vi "IQ_to_RF.vi"(7 "Header In":T1={"header info"={"Header"="", "Head length"=0}, "A/D info"={"# rf points per line"=0, "# lines per scan"=0, "sample rate MHz"=0, "# A/D bits"=0, "# bytes per A/D"=0, "TGC Flag"=0, "A/D Type"=""}, "Tranducer Info"={"bandwidth"=0.0, "center freq"=0.0, "start freq"=0.0, "ID"=0}, "Scan Info"={"delay"=0.0, "pivot distance"=0.0, "sector scan angle"=0.0, "operator"="", "Scan Mode"="", "location"=""}, "Time/Date Info"={"date"="", "time"=""}, "RF Info"={"RF file name"="", "RF file att"="", "RF cal file name"="", "RF cal file att"=""}, "Patient Info"={"ID"="", "extended ID"="", "age"=0, "sex"="", "previously\nscanned"="", "PSA"=0.0, "LOS"=1, "Ethnicty 2"=3, "Race"=3}, "Tissue Type"={"organ"=0, "disease type"=0, "disease location"=0, "IQ_pts"=0, "RcvBuffer"=0, "RcvFrame"=0, "IQBuff"=0, "IQFrame"=0, "IQPage"=0}, "Votage scaling"={"Digitizer (dB)"=0.0, "Gain (dB)"=0.0, "Atten (dB)"=0.0}, "Comment"="", "Misc Info"={"avg num"=0, "c speed"=0, "Div By or SF zones"=0, "XMIT CHS"=0, "RCV CHS"=0, "Xmit angle"=0.0}, "Therapy Parameters"={"Theraputic Freq (MHz)"=0.1, "Time on (s)"=1.0, "Therapy amplitude (mV)"=50.0, "Lines Before"=20, "Lines After"=80}, "Scan Settings"={"Energy (uJ or V)"=0, "Damp (Ohm) or Fc"=0, "HP Filt (KHz)"=0, "LP Filt (MHz)"=0, "Gain (db)"=0, "prf (kHz)"=0.0, "Distance between\nscan lines (um)"=0, "Distance between\nscan planes (um)"=0, "Scan line gap (um)"=0.0, "Scan plane gap (um)"=0.0}, "Compression Parameters"={"F1 (MHz)"=0.0, "F2 (MHz)"=0.0, "% taper"=0.0, "duration"=0.0}, "Patient Info Xtra"={"First Name"="", "Last Name"="", "Notes"=""}, "ROI Box"=[]} {"Compression Parameters"."% taper" min=50 max=1000 format="%.2f"; "Compression Parameters"."F2 (MHz)" format="%.3f"; "Compression Parameters"."F1 (MHz)" format="%.3f"; "Scan Settings"."prf (kHz)" format="%.2f"; "Therapy Parameters"."Therapy amplitude (mV)" min=50 max=1000 format="%.2f"; "Therapy Parameters"."Time on (s)" format="%.3f"; "Therapy Parameters"."Theraputic Freq (MHz)" format="%.3f"; "Patient Info"."Race" items=["Am Ind or Alaska", "Asian", "Hawaiian, Pac Isl", "Black or Afr Amer", "White", "more than one race", "unknown"]; "Patient Info"."Ethnicty 2" items=["Hispanic", "Non-Hispanic", "unknown"]; "Patient Info"."LOS" items=["1", "2", "3", "4", "5"]; "Patient Info"."PSA" format="%.1f"; "Scan Info"."delay" format="%.2f"; "Scan Info"."pivot distance" format="%.2f"; "Scan Info"."sector scan angle" format="%.2f"; "Tranducer Info"."bandwidth" format="%.2f"; "Tranducer Info"."center freq" format="%.2f"; "Tranducer Info"."start freq" format="%.2f"}, 9 "IQ Array In":i32[](array[numeric]), 11 "IQ Array":csg[][](array[numeric])) -> (0 "Z Out":csg[][](array[numeric]), 3 "RF Array":sgl[][](array[numeric]))   [LabVIEW 2022 SP3]
uses:
  Header.ctl
  <vilib>/Analysis/2dsp.llb/Rational Resample (single channel, DBL).vi
  <vilib>/Analysis/NI_AALPro.lvlib
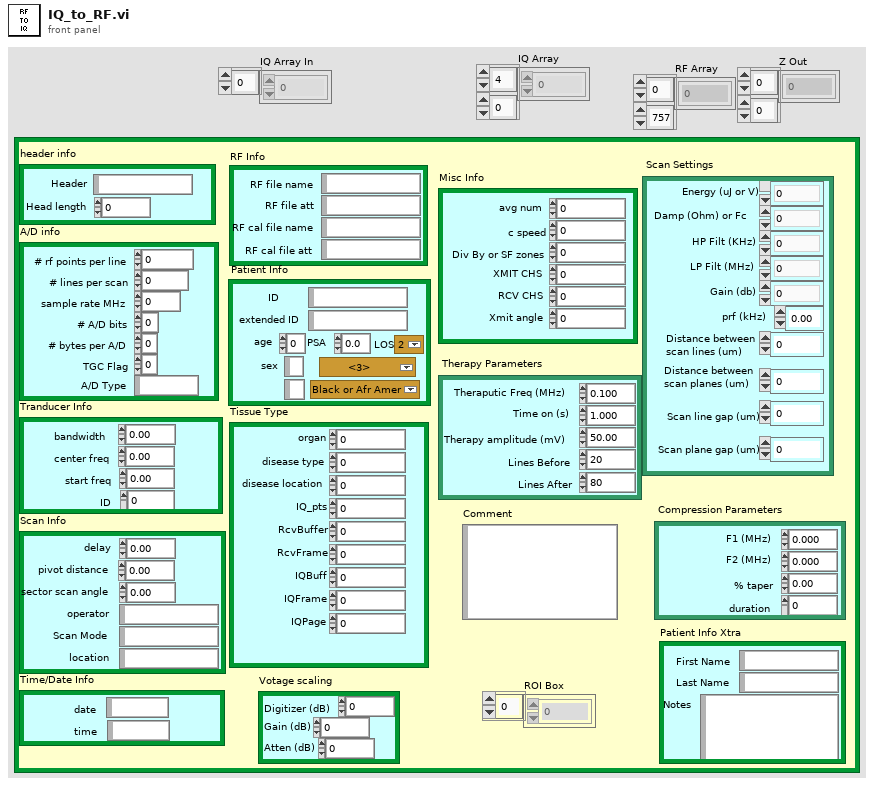
[diagram p1: front panel]
types:
  T1 = typedef "Header.ctl" = cluster{"header info":cluster{"Header":string, "Head length":i16}, "A/D info":cluster{"# rf points per line":u16, "# lines per scan":u16, "sample rate MHz":u16, "# A/D bits":i16, "# bytes per A/D":u16, "TGC Flag":u16, "A/D Type":string}, "Tranducer Info":cluster{"bandwidth":sgl, "center freq":sgl, "start freq":sgl, "ID":i32}, "Scan Info":cluster{"delay":sgl, "pivot distance":sgl, "sector scan angle":sgl, "operator":string, "Scan Mode":string, "location":string}, "Time/Date Info":cluster{"date":string, "time":string}, "RF Info":cluster{"RF file name":string, "RF file att":string, "RF cal file name":string, "RF cal file att":string}, "Patient Info":cluster{"ID":string, "extended ID":string, "age":u16, "sex":string, "previously\nscanned":string, "PSA":sgl, "LOS":u8, "Ethnicty 2":u8, "Race":u8}, "Tissue Type":cluster{"organ":i16, "disease type":i16, "disease location":i16, "IQ_pts":u16, "RcvBuffer":u8, "RcvFrame":u16, "IQBuff":u8, "IQFrame":u16, "IQPage":u8}, "Votage scaling":cluster{"Digitizer (dB)":sgl, "Gain (dB)":sgl, "Atten (dB)":sgl}, "Comment":string, "Misc Info":cluster{"avg num":u16, "c speed":i16, "Div By or SF zones":i16, "XMIT CHS":u8, "RCV CHS":u8, "Xmit angle":sgl}, "Therapy Parameters":cluster{"Theraputic Freq (MHz)":sgl, "Time on (s)":sgl, "Therapy amplitude (mV)":sgl, "Lines Before":u16, "Lines After":u16}, "Scan Settings":cluster{"Energy (uJ or V)":u8, "Damp (Ohm) or Fc":u8, "HP Filt (KHz)":u8, "LP Filt (MHz)":u8, "Gain (db)":u8, "prf (kHz)":sgl, "Distance between\nscan lines (um)":u16, "Distance between\nscan planes (um)":u16, "Scan line gap (um)":sgl, "Scan plane gap (um)":sgl}, "Compression Parameters":cluster{"F1 (MHz)":sgl, "F2 (MHz)":sgl, "% taper":sgl, "duration":sgl}, "Patient Info Xtra":cluster{"First Name":string, "Last Name":string, "Notes":string}, "ROI Box":u16[]}
  T2 = cluster{"alias rejection (dB)":dbl, "normalized bandwidth":dbl}
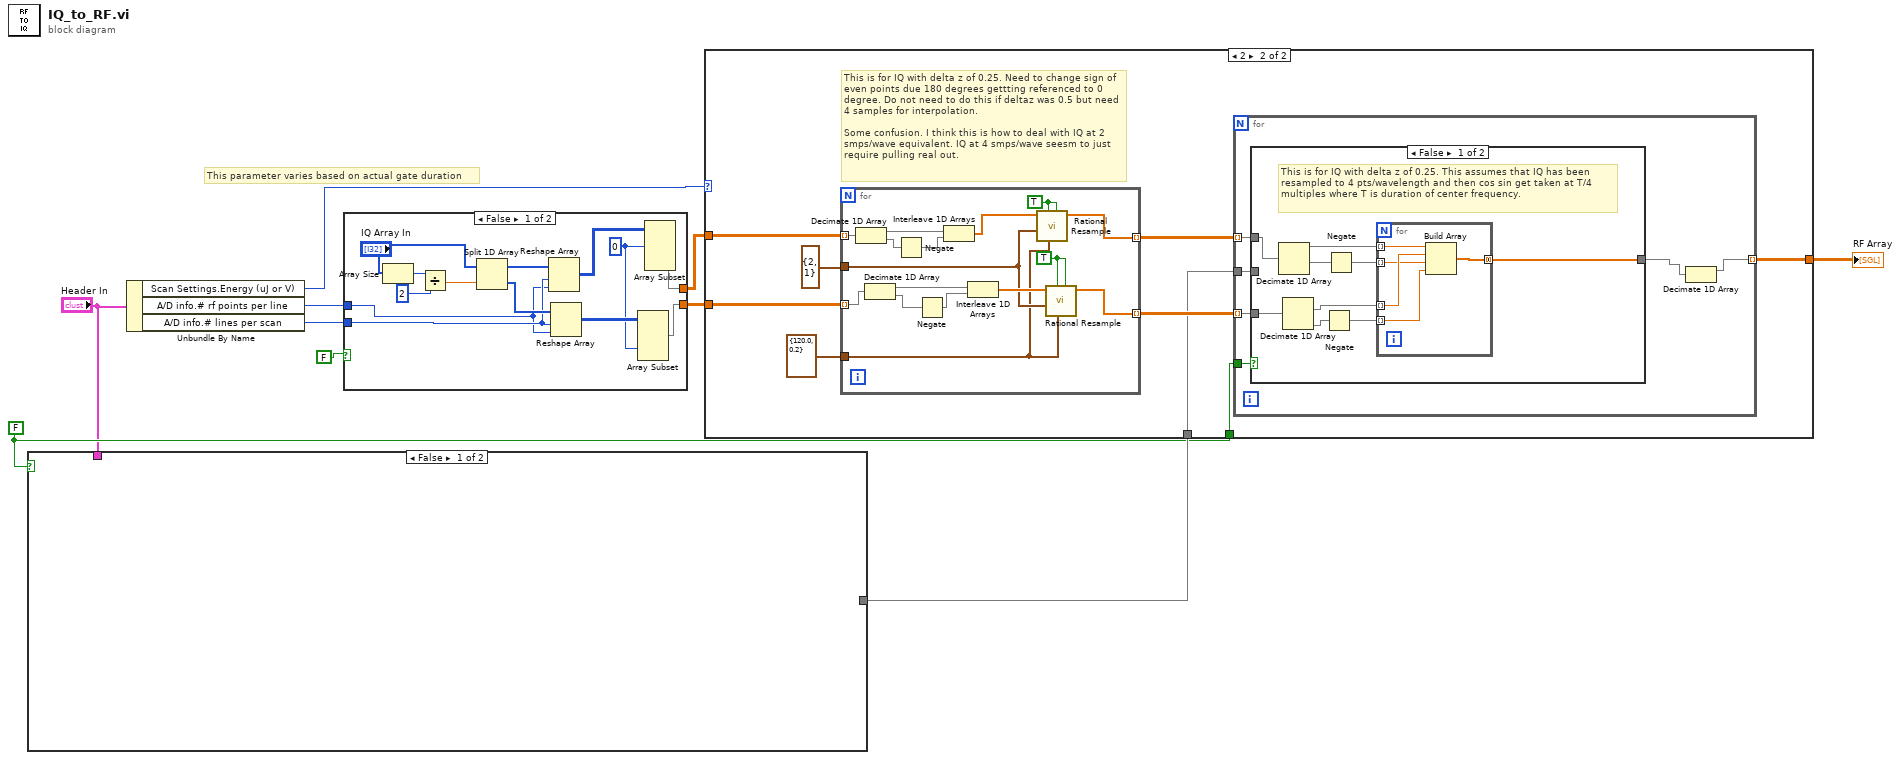
[diagram p0: block diagram]
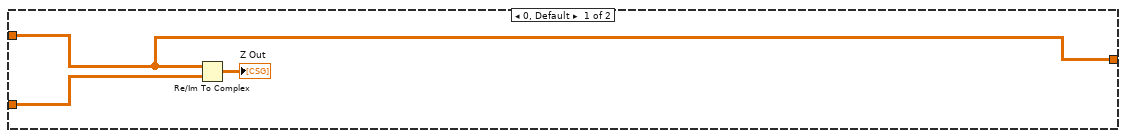
[diagram p2: hidden frame]
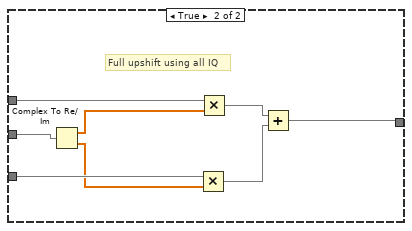
[diagram p3: hidden frame]
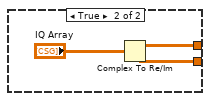
[diagram p4: hidden frame]
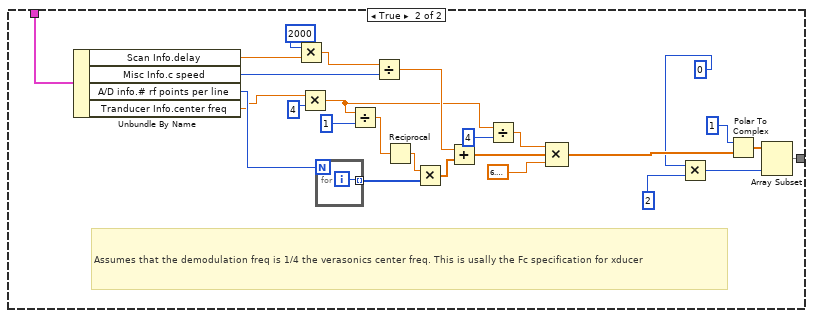
[diagram p5: hidden frame]
diagram:
  w9 = FALSE
  # "This parameter varies based on actual gate duration"
  n1 = case shown="False" w9 {
    tunnel: [_ w16] -> w10
    tunnel: "Header In" -> [_ w12]
    frame False {
    }
    frame True {
      # "Assumes that the demodulation freq is 1/4 the verasonics center freq. This is usally the Fc specification for xducer"
      n2 = Unbundle By Name(w12) -> ("Scan Info.delay"=w32:sgl, "Misc Info.c speed"=w29:i16, "A/D info.# rf points per line"=w33:u16, "Tranducer Info.center freq"=w15:sgl)
      n3 = Multiply(x=2000, y=w32) -> (x*y=w30:sgl)
      n4 = Multiply(x=w15, y=4) -> (x*y=w14:sgl)
      n5 = for {
        N: w33 -> [_]
        tunnel: [w37] -> w25 mode=indexing
        i -> [w37]
      }
      n6 = Divide(x=w14, y=1) -> (x/y=w24:sgl)
      n7 = Divide(x=w30, y=w29) -> (x/y=w28:sgl)
      n8 = Reciprocal(x=w24) -> (1/x=w23:sgl)
      n9 = Multiply(x=w23, y=w25) -> (x*y=w22:sgl[])
      n10 = Add(x=w28, y=w22) -> (x+y=w27:sgl[])
      n11 = Divide(x=w14, y=4) -> (x/y=w35:sgl)
      n12 = Compound Arithmetic op=MULTIPLY(w35, w27, 6.283185307179586) -> (w21:dbl[])
      n13 = Multiply(x=0 ("length"), y=2 ("upsampling factor")) -> (x*y=w17:i32)
      n14 = Polar To Complex(1:w21, 2:1 ("upsampling factor")) -> (0:w19:cdb[])
      n15 = Array Subset(array=w19, length=w17) -> (w16:cdb[])  [unwired: 1 in]
    }
  }
  n16 = Unbundle By Name("Header In") -> ("Scan Settings.Energy (uJ or V)"=w2:u8, "A/D info.# rf points per line"=w6:u16, "A/D info.# lines per scan"=w3:u16)
  n17 = case shown="False" FALSE {
    tunnel: w6 -> [w42 _]
    tunnel: [w46 w52] -> w5
    tunnel: [w44 w51] -> w4
    tunnel: w3 -> [w48 _]
    frame False {
      w43 = 0 ("index")
      n18 = Array Size(array="IQ Array In") -> (size(s)=w40:i32)
      n19 = Divide(x=w40, y=2) -> (x/y=w39:dbl)
      n20 = Split 1D Array(array="IQ Array In", index=w39) -> (first subarray=w50:i32[], second subarray=w49:i32[])
      n21 = Reshape Array(w50, w48, w42) -> (w47:i32[][])
      n22 = Reshape Array(w49, w48, w42) -> (w45:i32[][])
      n23 = Array Subset(array=w45, index (col)=w43) -> (w44:i32[][])  [unwired: 3 in]
      n24 = Array Subset(array=w47, index (col)=w43) -> (w46:i32[][])  [unwired: 3 in]
    }
    frame True {
      n25 = Complex To Re/Im(x + iy="IQ Array") -> (x=w52:sgl[][], y=w51:sgl[][])
    }
  }
  n26 = case shown="2" w2 {
    tunnel: w10 -> [_ w63]
    tunnel: w9 -> [_ w62]
    tunnel: w5 -> [w54 w61]
    tunnel: w4 -> [w56 w60]
    tunnel: [w54 w59] -> w1
    frame 0, Default {
      n27 = Re/Im To Complex(1:w56, 2:w54) -> (0:→"Z Out":csg[][])
    }
    frame 2 {
      # "This is for IQ with delta z of 0.25. Need to change sign of even points due 180 degrees gettting referenced to 0 degree. Do not need to do this if deltaz was 0.5 but need 4 samples for interpolation.\n\nSome confusion. I think this is how to deal with IQ at 2 smps/wave equivalent. IQ at 4 smps/wave seesm to just require pulling real out."
      n28 = for {
        tunnel: cluster{"interpolation":i32, "decimation":i32} {"interpolation"=2, "decimation"=1} ("resample factor") -> [w72]
        tunnel: w61 -> [w71] mode=indexing
        tunnel: w60 -> [w70] mode=indexing
        tunnel: T2 {"alias rejection (dB)"=120.0, "normalized bandwidth"=0.2} ("FIR filter specifications") -> [w69]
        tunnel: [w67] -> w65 mode=indexing
        tunnel: [w68] -> w64 mode=indexing
        w73 = TRUE ("anti-aliasing?")
        w78 = TRUE ("anti-aliasing?")
        n29 = Decimate 1D Array(w71) -> (w80:sgl[], w81:sgl[])
        n30 = Decimate 1D Array(w70) -> (w76:sgl[], w77:sgl[])
        n31 = Negate(x=w81) -> (-x=w79:sgl[])
        n32 = Negate(x=w77) -> (-x=w75:sgl[])
        n33 = Interleave 1D Arrays(w80, w79) -> (w66:sgl[])
        n34 = Interleave 1D Arrays(w76, w75) -> (w74:sgl[])
        n35 = call-poly <vilib>:"Rational Resample.vi"("anti-aliasing?"=w78, "FIR filter specifications"=w69, "reset"=w78, "resample factor"=w72, "X"=w66) -> ("Y"=w67:dbl[])  [unwired: 4 in, 2 out]
        n36 = call-poly <vilib>:"Rational Resample.vi"("anti-aliasing?"=w73, "FIR filter specifications"=w69, "reset"=w73, "resample factor"=w72, "X"=w74) -> ("Y"=w68:dbl[])  [unwired: 4 in, 2 out]
      }
      n37 = for {
        tunnel: [w82] -> w59 mode=indexing
        tunnel: w65 -> [w87] mode=indexing
        tunnel: w64 -> [w86] mode=indexing
        tunnel: w62 -> [w85]
        tunnel: w63 -> [w84]
        n38 = case shown="False" w85 {
          tunnel: [w93 w105] -> w83
          tunnel: w87 -> [w89 w109]
          tunnel: w86 -> [w88 w108]
          tunnel: w84 -> [_ w104]
          frame False {
            # "This is for IQ with delta z of 0.25. This assumes that IQ has been resampled to 4 pts/wavelength and then cos sin get taken at T/4 multiples where T is duration of center frequency."
            n39 = Decimate 1D Array(w89) -> (w96:dbl[], w92:dbl[])  [unwired: 2 out]
            n40 = Decimate 1D Array(w88) -> (w90:dbl[], w91:dbl[])  [unwired: 2 out]
            n41 = Negate(x=w91) -> (-x=w94:dbl[])
            n42 = Negate(x=w92) -> (-x=w95:dbl[])
            n43 = for {
              tunnel: w96 -> [w101] mode=indexing
              tunnel: w90 -> [w100] mode=indexing
              tunnel: w95 -> [w99] mode=indexing
              tunnel: w94 -> [w98] mode=indexing
              tunnel: [w97] -> w93 mode=concatenating
              n44 = Build Array(w101, w100, w99, w98) -> (w97:dbl[])
            }
          }
          frame True {
            # "Full upshift using all IQ"
            n45 = Complex To Re/Im(x + iy=w104) -> (x=w103:dbl[], y=w102:dbl[])
            n46 = Multiply(x=w108, y=w102) -> (x*y=w106:dbl[])
            n47 = Multiply(x=w109, y=w103) -> (x*y=w107:dbl[])
            n48 = Add(x=w107, y=w106) -> (x+y=w105:dbl[])
          }
        }
        n49 = Decimate 1D Array(w83) -> (w82:dbl[])  [unwired: 1 out]
      }
    }
  }
  "RF Array" <- w1
